vi "Constants.vi"() -> ()   [LabVIEW 2026, in "WebPage Addon Shared.lvlib"]
doc: "Use this Global VI to access the GUIDs assigned to the page resources of the Custom Device."
uses:
  WebPage Addon Shared.lvlib
panel:
  in  "Tab Control":enum32{"GUIDs", "Constants", "Properties"}(tab)=enum."Constants"
  in  "GUID.WebPageAddonDisable":string="5F723691-027A-41FF-9930-77045F19C5F0"
  in  "GUID.WebPageAddon":string="61c42cce-7210-4013-8cc7-f6e7840422ea"
  in  "Const.gRPCAddressFormat":string="%s:%d"
  in  "Const.WebAddressFormat":string="http://%s:%d"
  in  "Addon.Name":string="WebPage Addon"
  in  "Addon.Version":string="1.0.0"
  in  "Prop.HostedIP":string="Hosted IP"
  in  "Prop.gRPCPort":string="gRPC Port"
  in  "Prop.HostedPort":string="Hosted Port"
  in  "Prop.UpdateRate":string="Update Rate"
  in  "Compiled.Settings":string="Compiled.Settings"
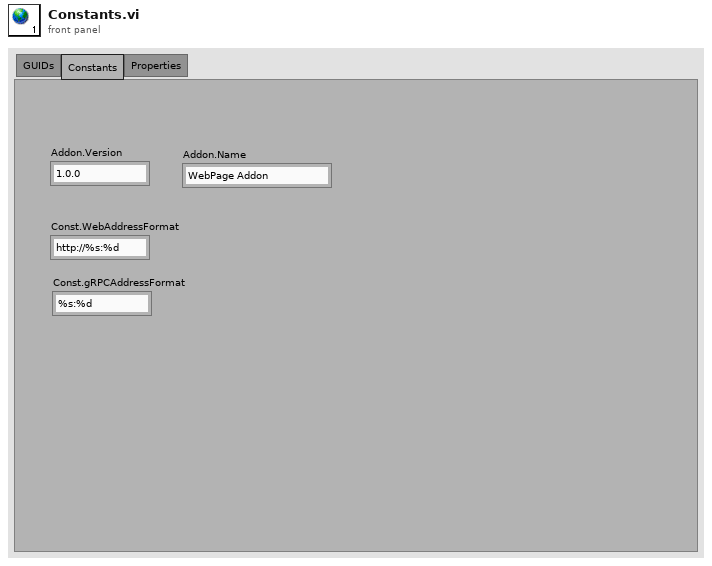
[diagram p1: front panel]
diagram:
